vi "Create URL.vi"(9 "endpoint":T1="v1/start-model", 10 "port":string(combo)="8080", 11 "Target IP Address":string="10.0.35.19") -> (3 "URL Out":string)   [LabVIEW 2020]
uses:
  Web Service/Endpoints.ctl
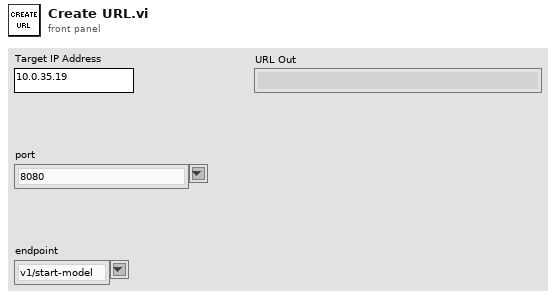
[diagram p1: front panel]
types:
  T1 = typedef "Endpoints.ctl" = string
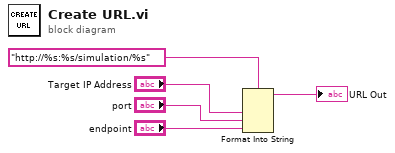
[diagram p0: block diagram]
diagram:
  n1 = Format Into String(format string="http://%s:%s/simulation/%s" ("url"), "Target IP Address", "port", "endpoint") -> (resulting string=→"URL Out":string)  [unwired: 2 in, 1 out]
